vi "List All Packages in SystemLink Repository.vi"(0 "SystemLink repo in":T1, 11 "error in (no error)":errorcluster) -> (4 "SystemLink repo out":T1, 8 "packages":string[][](table), 15 "error out":errorcluster)   [LabVIEW 2017, in "SystemLink_Repo_API.lvlib"]
doc: "Lists all the packages in the entire SystemLink repository.\n\nOutputs:\nPackages - This is a table (2D string array) that lists all the packages in the SystemLink repository. The table includes the name, version, filename, and package ID for each package."
uses:
  SystemLink_Repo_API.lvlib
  <vilib>/JDP Science/JSONtext/LVClass Serializer/JSONtext LVClass Serializer.lvclass
  <vilib>/httpClient/LabVIEWHTTPClient.lvlib
  73f63470-54eb-45b7-8baf-304f99d209d6.vi
  0c27402d-d134-44f2-9e9f-9c548188b8ee.vi
  <vilib>/httpClient/ClientHandle.ctl
  _support/systemlink repo.ctl
panel:
  out "body":string
  out "headers":string
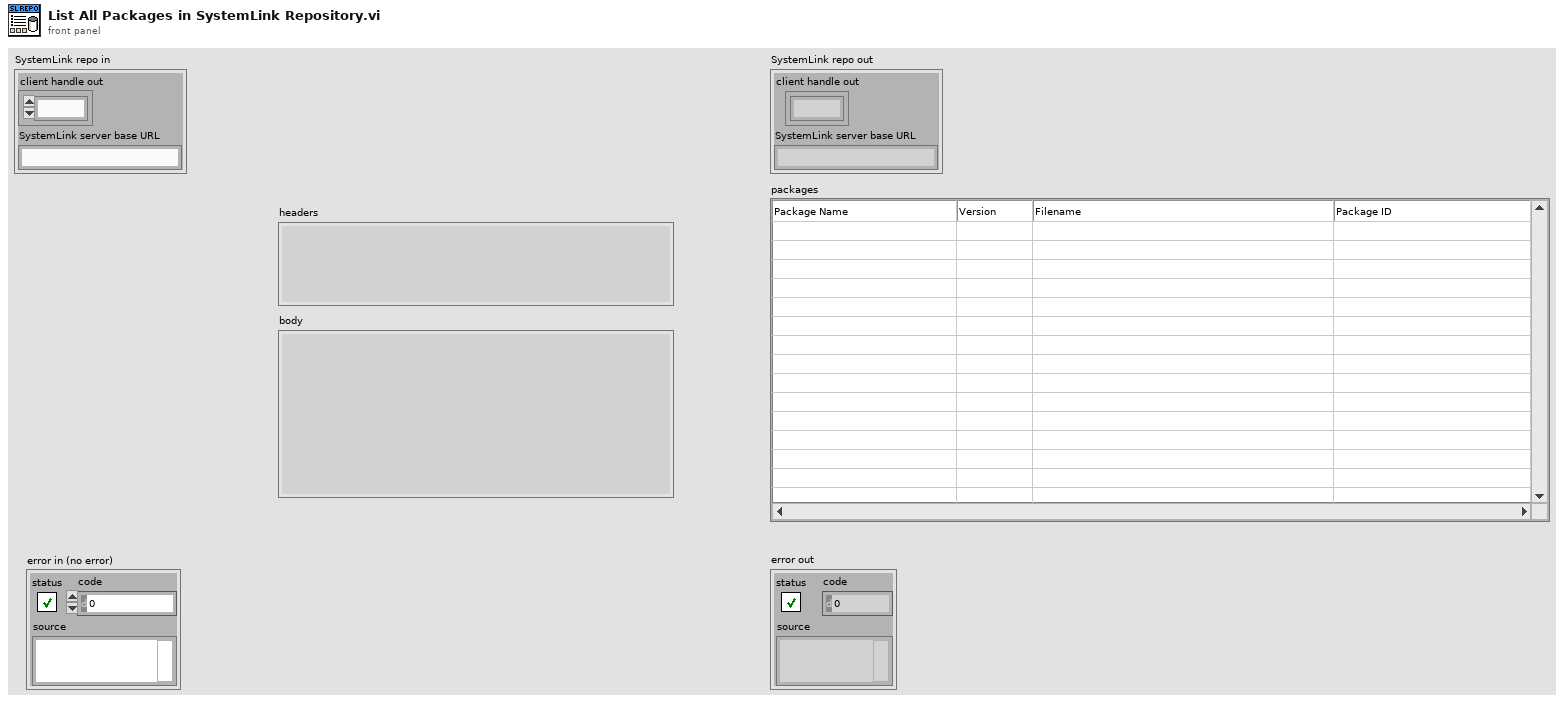
[diagram p1: front panel]
types:
  T1 = typedef "SystemLink_Repo_API.lvlib/systemlink repo.ctl" = cluster{"client handle out":T2, "SystemLink server base URL":string}
  T2 = typedef "LabVIEWHTTPClient.lvlib/ClientHandle.ctl" = refnum<k1>
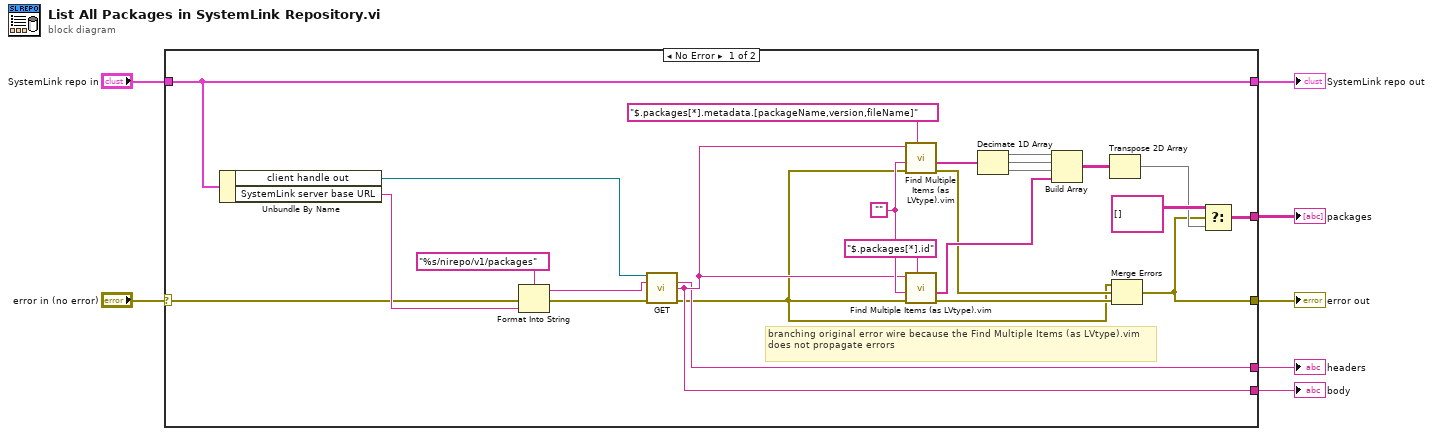
[diagram p0: block diagram]
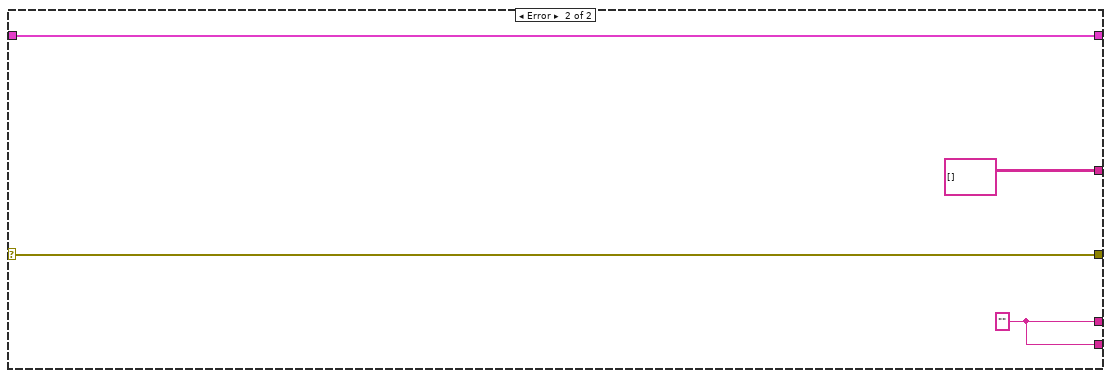
[diagram p2: hidden frame]
diagram:
  n1 = case shown="No Error" "error in (no error)" {
    selector: "error in (no error)" -> [w28 w36]
    tunnel: "SystemLink repo in" -> [w9 w33]
    tunnel: [w12 w36] -> w6
    tunnel: [w13 string[][] [] ("t")] -> w5
    tunnel: [w11 w34] -> w4
    tunnel: [w10 w34] -> w3
    tunnel: [w9 w33] -> w1
    frame No Error {
      w16 = ""
      # "branching original error wire because the Find Multiple Items (as LVtype).vim does not propagate errors"
      n2 = Unbundle By Name(w9) -> ("client handle out"=w30:T2, "SystemLink server base URL"=w29:string)
      n3 = Format Into String(format string="%s/nirepo/v1/packages", error in=w28, w29) -> (resulting string=w31:string, error out=w27:errorcluster)  [unwired: 1 in]
      n4 = call <vilib>:"GET.vi"("client handle"=w30, "url"=w31, "error in (no error)"=w27) -> ("headers"=w10:string, "body"=w11:string, "error out"=w8:errorcluster)  [unwired: 9 in, 1 out]
      n5 = call "Find Multiple Items (as LVtype).vim"("$Path or Item Name"="$.packages[*].metadata.[packageName,version,fileName]" ("$Path for packages 2"), "error in (no error)"=w8, "Data Type and Default Value"=w16, "JSON"=w11) -> ("error out"=w18:errorcluster, "Array of Data"=w23:string[])  [unwired: 4 in, 2 out]
      n6 = call "Find Multiple Items (as LVtype).vim"("$Path or Item Name"="$.packages[*].id" ("$Path for packages"), "error in (no error)"=w8, "Data Type and Default Value"=w16, "JSON"=w11) -> ("error out"=w17:errorcluster, "Array of Data"=w19:string[])  [unwired: 4 in, 2 out]
      n7 = Decimate 1D Array(w23) -> (w22:string[], w21:string[], w20:string[])
      n8 = Build Array(w22, w21, w20, w19) -> (w24:string[][])
      n9 = Transpose 2D Array(2D array=w24) -> (transposed array=w14:string[][])
      n10 = Merge Errors(w8, w18, w17) -> (w12:errorcluster)
      n11 = Select(t=string[][] [], s=w12, f=w14) -> (s? t:f=w13:string[][])
    }
    frame Error {
      w34 = "" ("headers")
    }
  }
  "error out" <- w6
  "SystemLink repo out" <- w1
  "packages" <- w5
  "headers" <- w3
  "body" <- w4
